vi "InitializeGPUandSLM.vi"(1 "TrueFrame":i32=3, 3 "deviceId":i32, 4 "Path to LUT file":path, 5 "SLM enabled":bool) -> (0 "CUDA/SLM error":errorcluster, 2 "return":i32)   [LabVIEW 2009]
uses:
  GenerateHologramCUDA.dll
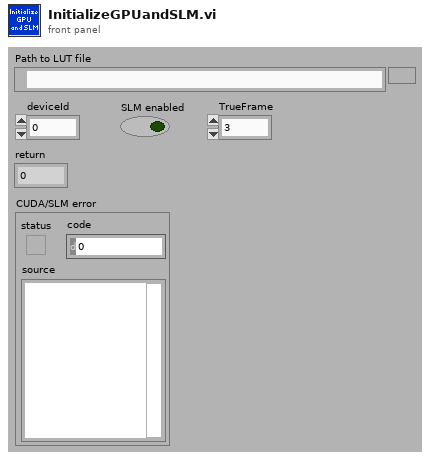
[diagram p1: front panel]
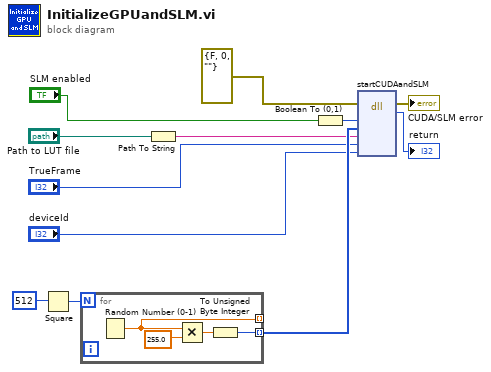
[diagram p0: block diagram]
diagram:
  n1 = Square(x=512 ("SLM size")) -> (x^2=w8:i32)
  n2 = for {
    N: w8 -> [_]
    tunnel: [w16] -> _ mode=indexing
    tunnel: [w13] -> w7 mode=indexing
    n3 = Random Number (0-1)() -> (number: 0 to 1=w16:dbl)
    n4 = Multiply(x=w16, y=255.0) -> (x*y=w14:dbl)
    n5 = To Unsigned Byte Integer(number=w14) -> (unsigned 8bit integer=w13:u8)
  }
  n6 = Path To String(path="Path to LUT file") -> (string=w2:string)
  n7 = Boolean To (0,1)(Boolean="SLM enabled") -> (0, 1=w10:i16)
  n8 = dll-call lib="C:/Users/Martin/Dropbox/GU/CUDA/GenerateHologramCUDA/LabVIEW/GenerateHologramCUDA.dll" fn="startCUDAandSLM"(error in=errorcluster {"status"=FALSE, "code"=0, "source"=""} ("CUDA/SLM error in (no error)"), "SLMenabled"=w10, "pSLMstart"=w7, "LUTpath"=w2, "TrueFrame"="TrueFrame", "deviceId"="deviceId") -> (error out=→"CUDA/SLM error":errorcluster, "return"=→"return":i32)  [unwired: 6 in, 2 out]
